vi "running average on cluster.vi"(7 "dt":dbl=0.2, 9 "x":dbl, 10 "t":dbl, 11 "averaging state cluster":T1) -> (3 "averaging state cluster out":T1)   [LabVIEW 2010]
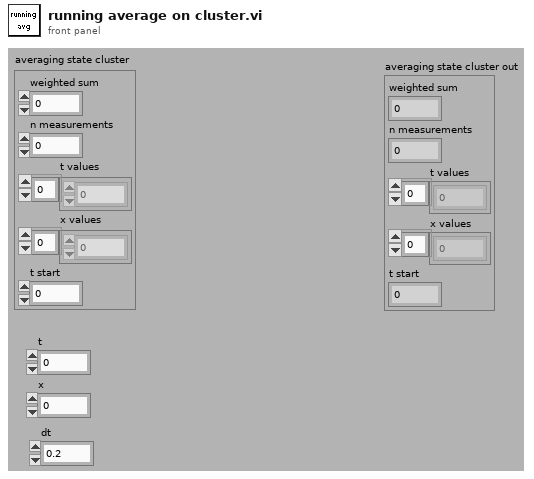
[diagram p1: front panel]
types:
  T1 = cluster{"weighted sum":dbl, "n measurements":dbl, "t values":dbl[], "x values":dbl[], "t start":dbl}
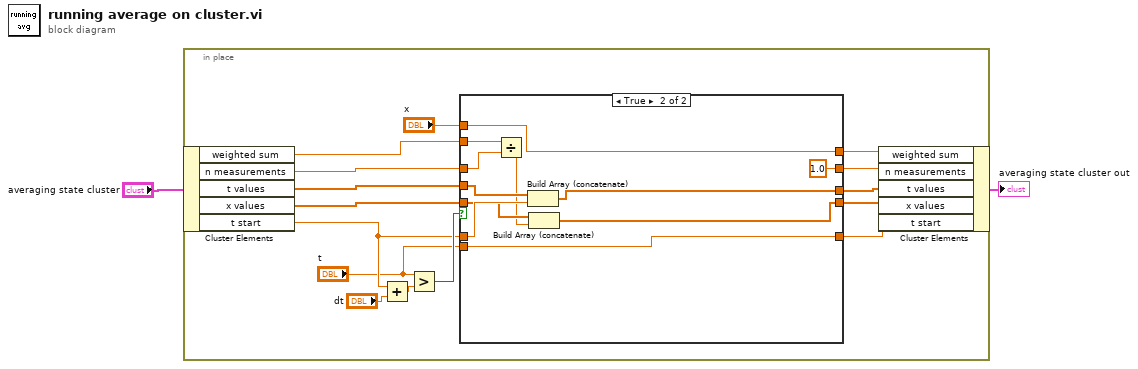
[diagram p0: block diagram]
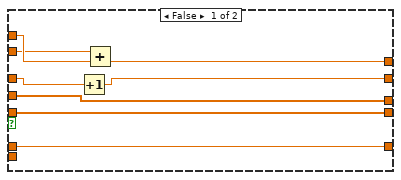
[diagram p2: hidden frame]
diagram:
  n1 = in-place {
    n2 = in-place-cluster #1("averaging state cluster") -> ("weighted sum"=w12:dbl, "n measurements"=w13:dbl, "t values"=w10:dbl[], "x values"=w8:dbl[], "t start"=w6:dbl)
    n3 = Add(x=w6, y="dt") -> (x+y=w17:dbl)
    n4 = Greater?(x="t", y=w17) -> (0:w16:bool)
    n5 = case shown="True" w16 {
      tunnel: "x" -> [w25 w35]
      tunnel: [w24 w35] -> w14
      tunnel: w13 -> [w22 w29]
      tunnel: w12 -> [w23 w30]
      tunnel: [w21 1.0] -> w11
      tunnel: w10 -> [w20 w33]
      tunnel: [w20 w31] -> w9
      tunnel: w8 -> [w19 w28]
      tunnel: [w19 w26] -> w7
      tunnel: w6 -> [w18 w32]
      tunnel: [w18 w36] -> w5
      tunnel: "t" -> [_ w36]
      frame False {
        n6 = Increment(x=w22) -> (x+1=w21:dbl)
        n7 = Add(x=w23, y=w25) -> (x+y=w24:dbl)
      }
      frame True {
        n8 = Divide(x=w30, y=w29) -> (x/y=w27:dbl)
        n9 = Build Array (concatenate)(w33, w32) -> (w31:dbl[])
        n10 = Build Array (concatenate)(w28, w27) -> (w26:dbl[])
      }
    }
    n11 = in-place-cluster #1("weighted sum"=w14, "n measurements"=w11, "t values"=w9, "x values"=w7, "t start"=w5) -> (→"averaging state cluster out":T1)
  }
